vi "Hash-string.vi"(7 "HASH-method":T1=enum."SHA-256" caption="HASH-method (SHA-256)", 8 "error in (no error)":errorcluster, 11 "Message":string="The quick brown fox jumps over the lazy dog") -> (0 "error out":errorcluster, 1 "ASCII formatted hash":string, 3 "binary string hash":string caption="binary string (hex formatted)")   [LabVIEW 2012, in "Encryption.lvlib"]
doc: "Calculates a hash for the given <b>Message</b>.\n\n(c) Ton Plomp, 2011\nTHIS SOFTWARE IS PROVIDED AS IS, AND ANY WARRANTY IS REJECTED"
uses:
  Encryption.lvlib
  hash-types.ctl
  Sub/SHA-2_U32_types.ctl
  Sub/SHA-2_U64_types.ctl
  <userlib>/_OpenG.lib/md5/md5.llb/MD5 Message Digest (Binary String)__ogtk.vi
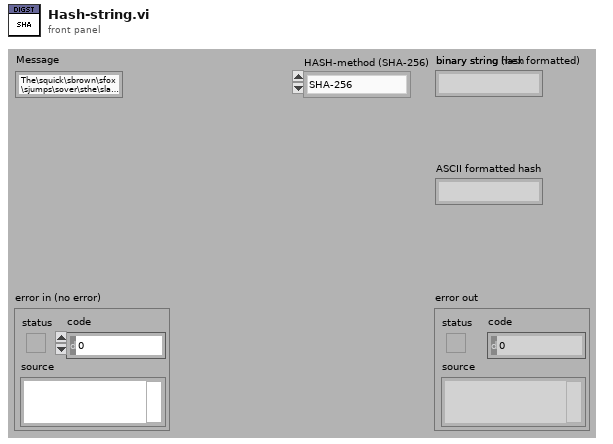
[diagram p1: front panel]
types:
  T1 = typedef "Encryption.lvlib/hash-types.ctl" = enum16{"MD5", "SHA-1", "SHA-224", "SHA-256", "SHA-384", "SHA-512"}
  T2 = typedef "Encryption.lvlib/SHA-2_U32_types.ctl" = enum16{"256", "224"}
  T3 = typedef "Encryption.lvlib/SHA-2_U64_types.ctl" = enum16{"512", "384"}
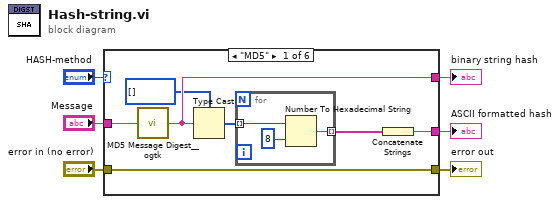
[diagram p0: block diagram]
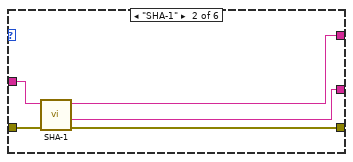
[diagram p2: hidden frame]
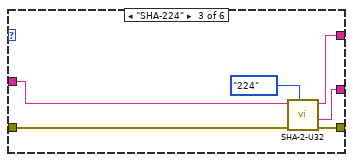
[diagram p3: hidden frame]
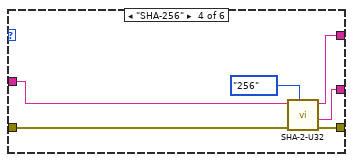
[diagram p4: hidden frame]
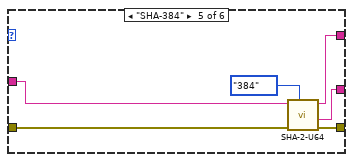
[diagram p5: hidden frame]
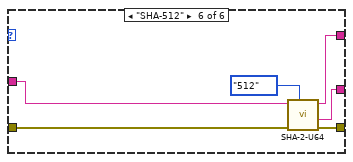
[diagram p6: hidden frame]
diagram:
  n1 = case shown="\"MD5\"" "HASH-method" {
    tunnel: "Message" -> [w13 w21 w27 w33 w39 w45]
    tunnel: [w8 w20 w26 w32 w38 w44] -> w4
    tunnel: "error in (no error)" -> [w8 w19 w25 w31 w37 w43]
    tunnel: [w10 w18 w24 w30 w36 w42] -> w2
    tunnel: [w9 w17 w23 w29 w35 w41] -> w1
    frame "MD5" {
      n2 = call-poly <userlib>:"MD5 Message Digest__ogtk.vi"("Message"=w13) -> ("MD5 Message Digest"=w10:string)
      n3 = Type Cast(type=u32[] [], x=w10) -> (*(type *) &x=w11:u32[])
      n4 = for {
        tunnel: w11 -> [w16] mode=indexing
        tunnel: [w14] -> w12 mode=indexing
        n5 = Number To Hexadecimal String(1:i16 8 ("width (-)"), 2:w16) -> (0:w14:string)
      }
      n6 = Concatenate Strings(w12) -> (w9:string)
    }
    frame "SHA-1" {
      n7 = call "SHA-1.vi"("error in (no error)"=w19, "Message"=w21) -> ("error out"=w20:errorcluster, "ASCII Formatted hash"=w17:string, "binary string hash"=w18:string)  [unwired: 7 in]
    }
    frame "SHA-224" {
      n8 = call "SHA-2-U32.vi"("Type"=SHA-2_U32_types."224", "error in (no error)"=w25, "Message"=w27) -> ("error out"=w26:errorcluster, "ASCII formatted hash"=w23:string, "binary string hash"=w24:string)  [unwired: 6 in]
    }
    frame "SHA-256" {
      n9 = call "SHA-2-U32.vi"("Type"=SHA-2_U32_types."256", "error in (no error)"=w31, "Message"=w33) -> ("error out"=w32:errorcluster, "ASCII formatted hash"=w29:string, "binary string hash"=w30:string)  [unwired: 6 in]
    }
    frame "SHA-384" {
      n10 = call "SHA-2-U64.vi"("Type"=SHA-2_U64_types."384", "error in (no error)"=w37, "Message"=w39) -> ("error out"=w38:errorcluster, "ASCII Formatted hash"=w35:string, "binary string hash"=w36:string)  [unwired: 6 in]
    }
    frame "SHA-512" {
      n11 = call "SHA-2-U64.vi"("Type"=SHA-2_U64_types."512", "error in (no error)"=w43, "Message"=w45) -> ("error out"=w44:errorcluster, "ASCII Formatted hash"=w41:string, "binary string hash"=w42:string)  [unwired: 6 in]
    }
  }
  "error out" <- w4
  "binary string hash" <- w2
  "ASCII formatted hash" <- w1
